vi "Sistema_de_Nivel.vi"() -> ()   [LabVIEW 2014]
panel:
  out "Knob 2":dbl=2255.47371276242
  in  "PARADA DE EMERGENCIA":bool
  out "Medidor de Llenado Tanque Principal":dbl(knob) scale=0.0..1000.0
  in  "Caudal de Llenado \nUV/Seg":dbl(knob)=46.98903568255046 scale=0.0..100.0
  out "Nivel Mínimo\nTanque Secundario":bool
  out "Nivel Máximo\nTanque Secuandario":bool
  out "Nivel Mínimo \nAlcanzado\nTanque Principal":bool
  out "Nivel Máximo \nAlcanzado\nTanque Principal":bool
  out "Medidor de Llenado Tanque Secundario":dbl(knob) scale=0.0..1800.0
  out "TANQUE DE LLENADO SECUNDARIO":dbl(slide) scale=0.0..1800.0 scale format="%#_5g"
  in  "Nivel Mínimo T2":dbl(slide) scale=0.0..1800.0 scale format="%#_5g"
  in  "Nivel  Máximo T2":dbl(slide)=1400.9433962264152 scale=0.0..1800.0 scale format="%#_5g"
  out "TANQUE DE LLENADO PRINCIPAL":dbl(slide) scale=0.0..1000.0
  in  "Nivel \nMínimo":dbl(slide)=60.24096385542169 scale=0.0..1000.0 scale format="%#_5g"
  in  "Nivel \nMáximo":dbl(slide)=853.1746031746032 scale=0.0..1000.0
  # "UNIVERSIDAD DE ORIENTE NÚCLEO MONAGAS\nESCUELA DE INGENIERÍA DE SISTEMAS\nASIGNATURA SISTEMAS DINÁMICOS\nMATURIN/MONAGAS/VENEZUELA"
  # "REALIZADO POR:\nCARROZZA CARLOS C.I: 21.050.636\nVIANI NILSO C.I: 20.740.569"
  # "PROFESOR:\nING. MARCOS RODRÍGUEZ"
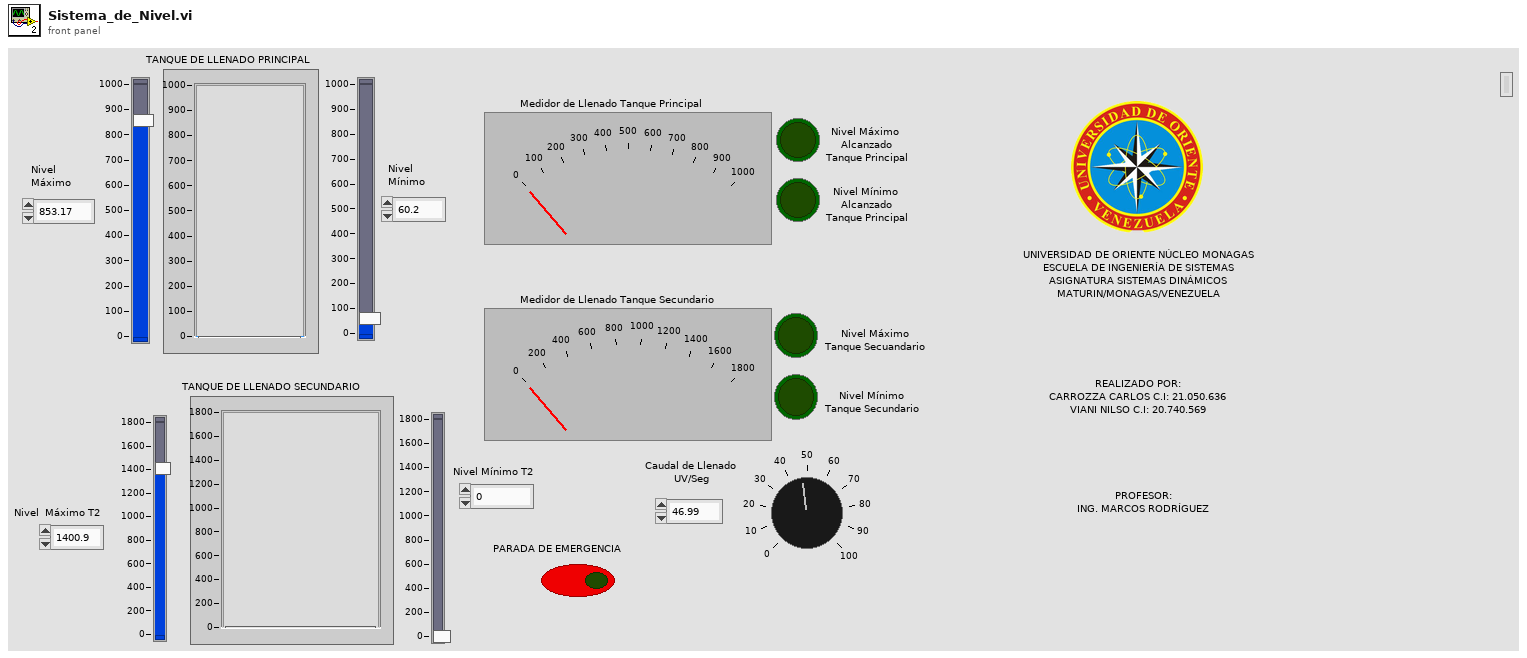
[diagram p1: front panel]
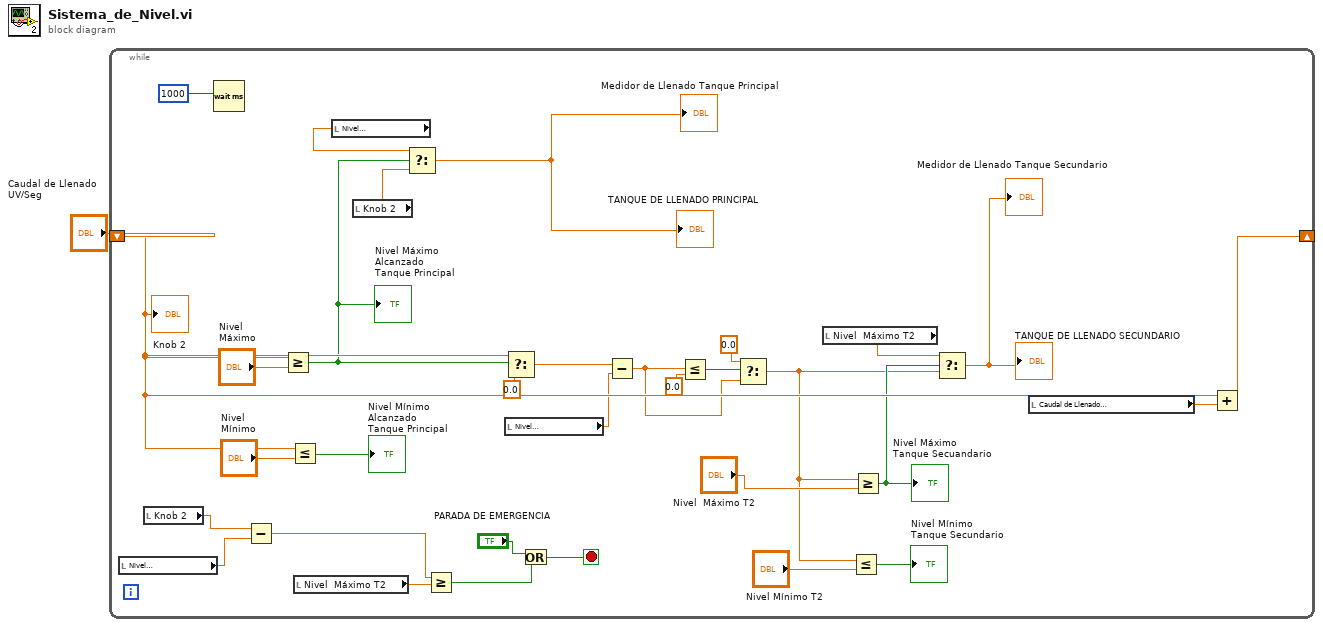
[diagram p0: block diagram]
diagram:
  n1 = while {
    shift-right: [w28] -> _
    shift-left: "Caudal de Llenado \nUV/Seg" -> [w22]
    stop <- w8 stop-if-true
    n2 = local read "Nivel \nMáximo"() -> (w3:dbl)
    n3 = local read "Knob 2"() -> (w4:dbl)
    n4 = Wait (ms)(milliseconds to wait=u32 1000) -> ()  [unwired: 1 out]
    n5 = Subtract(x=w4, y=w3) -> (x-y=w2:dbl)
    n6 = Greater Or Equal?(x=w22, y="Nivel \nMáximo") -> (x >= y?=w10:bool)
    "Nivel Máximo \nAlcanzado\nTanque Principal" <- w10
    n7 = Less Or Equal?(x=w22, y="Nivel \nMínimo") -> (x <= y?=→"Nivel Mínimo \nAlcanzado\nTanque Principal":bool)
    n8 = local read "Nivel  Máximo T2"() -> (w5:dbl)
    n9 = local read "Nivel \nMáximo"() -> (w25:dbl)
    n10 = local read "Knob 2"() -> (w24:dbl)
    n11 = Select(t=w25, s=w10, f=w24) -> (s? t:f=→"TANQUE DE LLENADO PRINCIPAL" →"Medidor de Llenado Tanque Principal":dbl)
    n12 = Greater Or Equal?(x=w2, y=w5) -> (x >= y?=w6:bool)
    n13 = local read "Nivel \nMáximo"() -> (w20:dbl)
    n14 = Select(t=w22, s=w10, f=0.0) -> (s? t:f=w21:dbl)
    n15 = Or(x="PARADA DE EMERGENCIA", y=w6) -> (x .or. y?=w8:bool)
    n16 = Subtract(x=w21, y=w20) -> (x-y=w16:dbl)
    n17 = Less Or Equal?(x=w16, y=0.0) -> (x <= y?=w18:bool)
    n18 = Select(t=0.0, s=w18, f=w16) -> (s? t:f=w13:dbl)
    n19 = local read "Nivel  Máximo T2"() -> (w12:dbl)
    n20 = Less Or Equal?(x=w13, y="Nivel Mínimo T2") -> (x <= y?=→"Nivel Mínimo\nTanque Secundario":bool)
    n21 = Greater Or Equal?(x=w13, y="Nivel  Máximo T2") -> (x >= y?=w14:bool)
    "Nivel Máximo\nTanque Secuandario" <- w14
    n22 = Select(t=w12, s=w14, f=w13) -> (s? t:f=→"Medidor de Llenado Tanque Secundario" →"TANQUE DE LLENADO SECUNDARIO":dbl)
    n23 = local read "Caudal de Llenado \nUV/Seg"() -> (w26:dbl)
    n24 = Add(x=w22, y=w26) -> (x+y=w28:dbl)
    "Knob 2" <- w22
  }
